vi "numArray2String.vi"(1 "输入数组":dbl[](array[numeric]) format="%_6g") -> (0 "输出字符串":string)   [LabVIEW 2018]
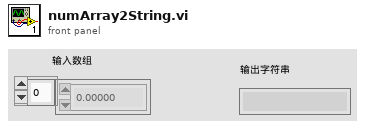
[diagram p1: front panel]
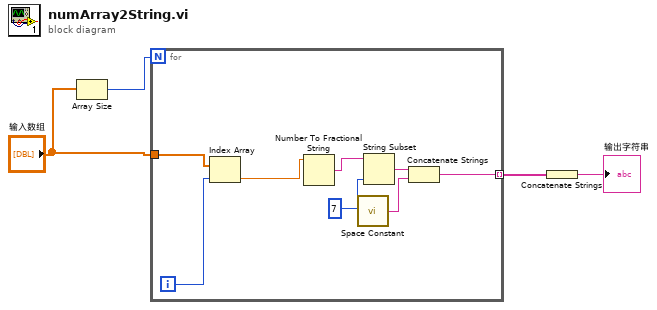
[diagram p0: block diagram]
diagram:
  n1 = Array Size(array="输入数组") -> (size(s)=w4:i32)
  n2 = for {
    N: w4 -> [_]
    tunnel: "输入数组" -> [w12]
    tunnel: [w8] -> w2 mode=indexing
    i -> [w11]
    n3 = Index Array(array=w12, index=w11) -> (element=w10:dbl)
    n4 = Number To Fractional String(number=w10) -> (F-format string=w6:string)  [unwired: 3 in]
    n5 = call <vilib>:"Space Constant.vi"() -> ("String"=w9:string)
    n6 = String Subset(string=w6, length (rest)=7) -> (substring=w7:string)  [unwired: 1 in]
    n7 = Concatenate Strings(w7, w9) -> (w8:string)
  }
  n8 = Concatenate Strings ("连接字符串")(w2) -> (→"输出字符串":string)
